vi "UDP_read_integer.vi"() -> ()   [LabVIEW 2014]
panel:
  in  "stop":bool
  out "Numeric":dbl
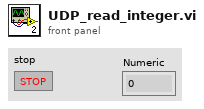
[diagram p1: front panel]
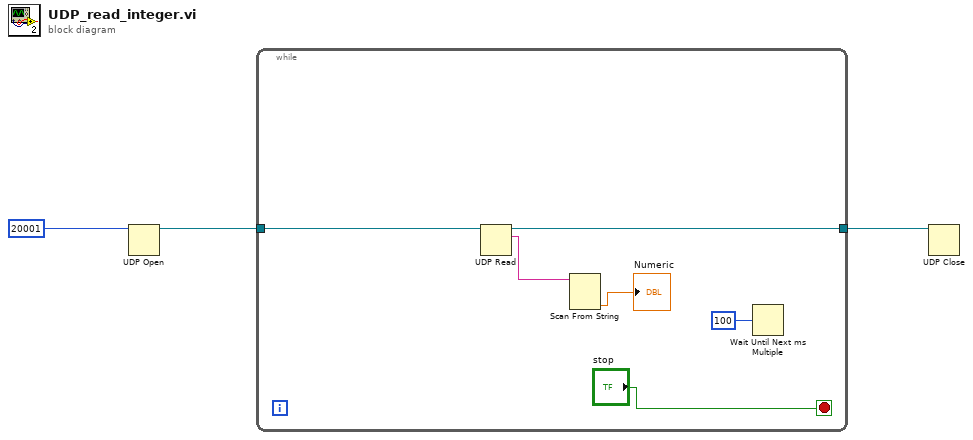
[diagram p0: block diagram]
diagram:
  n1 = UDP Open(11:u16 20001 ("port")) -> (port=w2:refnum<k16>)  [unwired: 4 in, 2 out]
  n2 = while {
    tunnel: w2 -> [w9]
    tunnel: [w8] -> w1
    stop <- "stop" stop-if-true
    n3 = UDP Read(connection ID=w9) -> (data out=w5:string, 3:w8:refnum<k16>)  [unwired: 3 in, 3 out]
    n4 = Scan From String(input string=w5) -> (output 1=→"Numeric":dbl)  [unwired: 4 in, 3 out]
    n5 = Wait Until Next ms Multiple(millisecond multiple=u32 100) -> ()  [unwired: 1 out]
  }
  n6 = UDP Close(connection ID=w1) -> ()  [unwired: 1 in, 2 out]
